vi "PM5000_SagSwell_Alarmas_DEMO.vi"() -> (14 "PQ_Alarmas":bool[](array[boolean]), 15 "PQ_Alarmas 2":bool[](array[boolean]), 16 "PQ_Alarmas 3":bool[](array[boolean]), 17 "PQ_Alarmas 4":bool[](array[boolean]), 18 "PQ_Alarmas 5":bool[](array[boolean]), 19 "PQ_Alarmas 6":bool[](array[boolean]))   [LabVIEW 2018]
doc: "Lee la tabla de memoria RealTime_VIF_Power del equipo PowerMonitor 5000, ademas filtra y ordena las variables de interez de la tabla de memoria.\n\nLee las siguientes variables de la tabla RealTime_VIF_Power:\n\n*V1_V2_Volts\n*V2_V3_Volts\n*V3_V1_Volts\n*I1_Amps\n*I2_Amps\n*I3_Amps\n*Frequency_Hz\n*Total_kW\n*Total_kVAR\n*Total_kVA\n*Total_True_PF\n*Total_Disp_PF"
panel:
  in  "TRANSIENTE 6":bool
  in  "SWELL 6":bool
  in  "SAG 6":bool
  in  "TRANSIENTE 5":bool
  in  "SWELL 5":bool
  in  "SAG 5":bool
  in  "TRANSIENTE 4":bool
  in  "SWELL 4":bool
  in  "SAG 4":bool
  in  "TRANSIENTE 3":bool
  in  "SWELL 3":bool
  in  "SAG 3":bool
  in  "TRANSIENTE 2":bool
  in  "SWELL 2":bool
  in  "SAG 2":bool
  in  "ID_EQUIPO":i32=1
  in  "TRANSIENTE":bool
  in  "SWELL":bool
  in  "SAG":bool
  # "GENERADOR 1"
  # "GENERADOR 2"
  # "GENERADOR 3"
  # "GENERADOR 4"
  # "GENERADOR 5"
  # "GENERADOR 2"
  # "Sag"
  # "Sag"
  # "Sag"
  # "Sag"
  # "Sag"
  # "Sag"
  # "Swell"
  # "Swell"
  # "Swell"
  # "Swell"
  # "Swell"
  # "Swell"
  # "Transient"
  # "Transient"
  # "Transient"
  # "Transient"
  # "Transient"
  # "Transient"
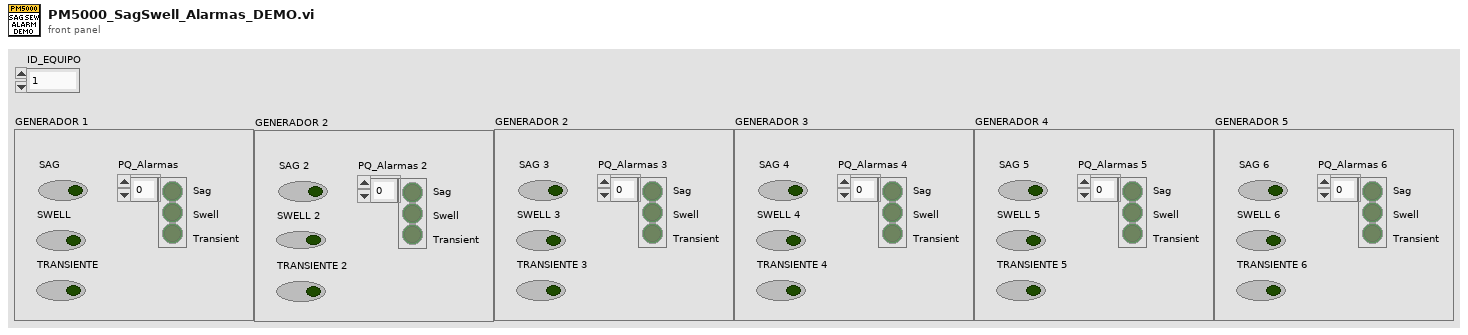
[diagram p1: front panel]
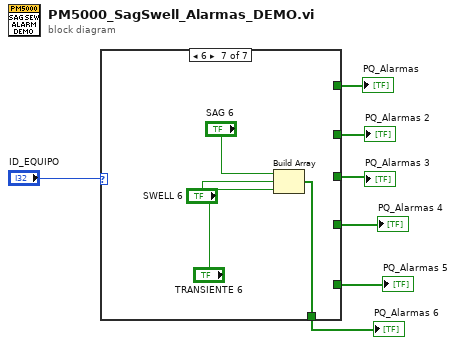
[diagram p0: block diagram]
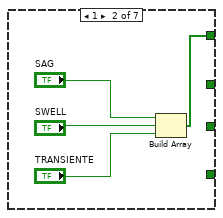
[diagram p3: hidden frame]
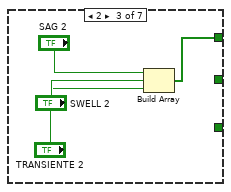
[diagram p4: hidden frame]
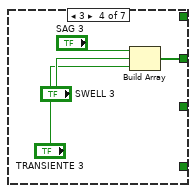
[diagram p5: hidden frame]
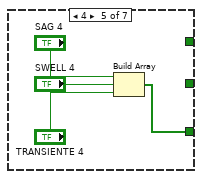
[diagram p6: hidden frame]
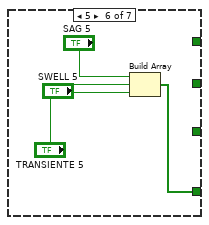
[diagram p7: hidden frame]
diagram:
  n1 = case shown="6" "ID_EQUIPO" {
    tunnel: [_ w8 _ _ _ _ _] -> w6
    tunnel: [_ _ w12 _ _ _ _] -> w5
    tunnel: [_ _ _ w16 _ _ _] -> w4
    tunnel: [_ _ _ _ w20 _ _] -> w3
    tunnel: [_ _ _ _ _ w24 _] -> w2
    tunnel: [_ _ _ _ _ _ w28] -> w1
    frame 0, Default {
    }
    frame 1 {
      n2 = Build Array("SAG", "SWELL", "TRANSIENTE") -> (w8:bool[])
    }
    frame 2 {
      n3 = Build Array("SAG 2", "SWELL 2", "TRANSIENTE 2") -> (w12:bool[])
    }
    frame 3 {
      n4 = Build Array("SAG 3", "SWELL 3", "TRANSIENTE 3") -> (w16:bool[])
    }
    frame 4 {
      n5 = Build Array("SAG 4", "SWELL 4", "TRANSIENTE 4") -> (w20:bool[])
    }
    frame 5 {
      n6 = Build Array("SAG 5", "SWELL 5", "TRANSIENTE 5") -> (w24:bool[])
    }
    frame 6 {
      n7 = Build Array("SAG 6", "SWELL 6", "TRANSIENTE 6") -> (w28:bool[])
    }
  }
  "PQ_Alarmas" <- w6
  "PQ_Alarmas 2" <- w5
  "PQ_Alarmas 3" <- w4
  "PQ_Alarmas 4" <- w3
  "PQ_Alarmas 5" <- w2
  "PQ_Alarmas 6" <- w1
